vi "XY Graph Show-Hide Grid.vi"(8 "Error In":errorcluster, 9 "Hide (F) /Show (T)":bool, 11 "XYGraph Ref":T1) -> (0 "Error Out":errorcluster, 1 "Grid Shown?":bool, 3 "XYGraph Ref out":T1)   [LabVIEW 2021, in "XY Graph Add-Ons.lvlib"]
uses:
  XY Graph Add-Ons.lvlib
  XY Graph Refnum.ctl
  <vilib>/Utility/miscctls.llb/LVMajorAndMinorColorsTypeDef.ctl
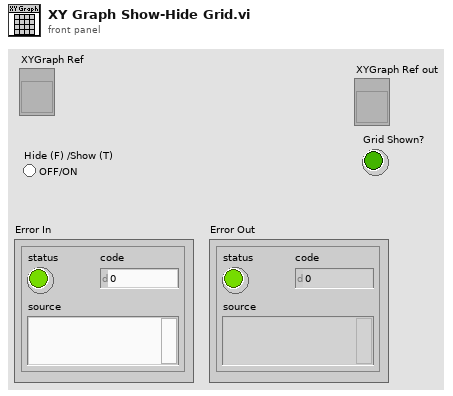
[diagram p1: front panel]
types:
  T1 = typedef "XY Graph Add-Ons.lvlib/XY Graph Refnum.ctl" = refnum<vi>
  T2 = typedef "LVMajorAndMinorColorsTypeDef.ctl" = cluster{"Major Color":u32, "Minor Color":u32}
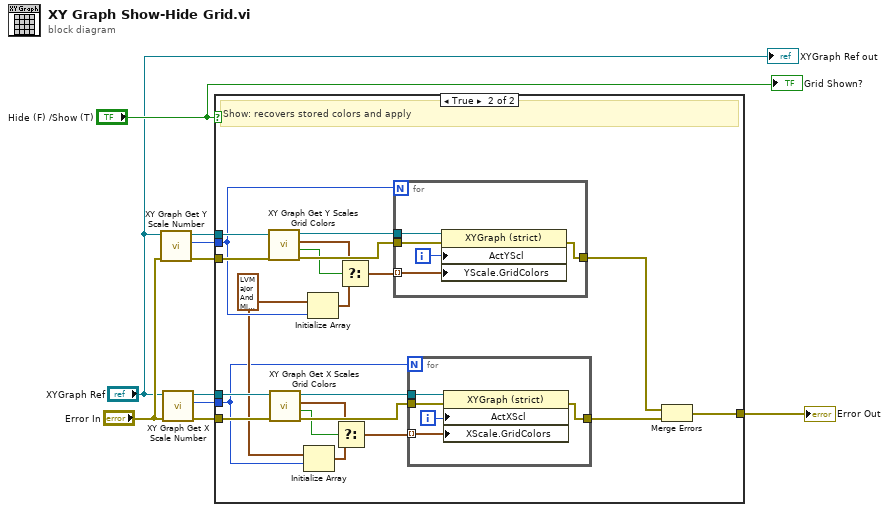
[diagram p0: block diagram]
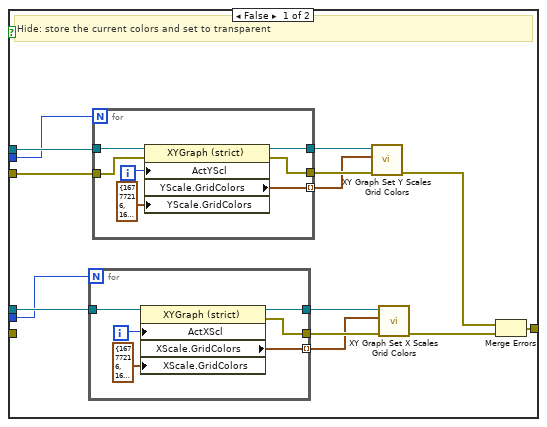
[diagram p2: hidden frame]
diagram:
  n1 = call "XY Graph Get Y Scale Number.vi"("Error In"="Error In", "XYGraph Ref"="XYGraph Ref") -> ("Error Out"=w3:errorcluster, "# Y Scales"=w2:i32, "XYGraph Ref out"=w4:T1)  [unwired: 7 in]
  n2 = call "XY Graph Get X Scale Number.vi"("Error In"="Error In", "XYGraph Ref"="XYGraph Ref") -> ("Error Out"=w7:errorcluster, "# X Scales"=w5:i32, "XYGraph Ref out"=w6:T1)  [unwired: 7 in]
  n3 = case shown="True" "Hide (F) /Show (T)" {
    tunnel: w6 -> [w24 w53]
    tunnel: [w16 w51] -> w10
    tunnel: w7 -> [_ w54]
    tunnel: w5 -> [w11 w39]
    tunnel: w4 -> [w14 w52]
    tunnel: w3 -> [w13 w49]
    tunnel: w2 -> [w12 w45]
    frame False {
      # "Hide: store the current colors and set to transparent"
      n4 = for {
        N: w11 -> [_]
        tunnel: [w34] -> w22 mode=indexing
        tunnel: [w36] -> w23
        tunnel: w24 -> [w37]
        tunnel: [w35] -> w21
        i -> [w32]
        n5 = property class="XYGraph (strict)"(reference=w37, "ActXScl"=w32, "XScale.GridColors"=cluster{"Major Color":u32, "Minor Color":u32} {"Major Color"=16777216, "Minor Color"=16777216} ("X Scale.Grid Colors")) -> (reference out=w35:T1, error out=w36:errorcluster, "XScale.GridColors"=w34:T2)  [unwired: 1 in]
      }
      n6 = for {
        N: w12 -> [_]
        tunnel: [w27] -> w18 mode=indexing
        tunnel: w13 -> [w30]
        tunnel: [w29] -> w19
        tunnel: w14 -> [w31]
        tunnel: [w28] -> w20
        i -> [w25]
        n7 = property class="XYGraph (strict)"(reference=w31, error in=w30, "ActYScl"=w25, "YScale.GridColors"=cluster{"Major Color":u32, "Minor Color":u32} {"Major Color"=16777216, "Minor Color"=16777216} ("X Scale.Grid Colors")) -> (reference out=w28:T1, error out=w29:errorcluster, "YScale.GridColors"=w27:T2)
      }
      n8 = call "XY Graph Set Y Scales Grid Colors.vi"("error in (no error)"=w19, "Array of Grid Colors"=w18, "XYGraph in"=w20) -> ("error out"=w17:errorcluster)  [unwired: 7 in, 1 out]
      n9 = call "XY Graph Set X Scales Grid Colors.vi"("error in (no error)"=w23, "Array of Grid Colors"=w22, "XYGraph in"=w21) -> ("error out"=w15:errorcluster)  [unwired: 7 in, 1 out]
      n10 = Merge Errors(w17, w15) -> (w16:errorcluster)
    }
    frame True {
      w40 = T2 {"Major Color"=13816530, "Minor Color"=13816530} ("Y Scale.Grid Colors")
      # "Show: recovers stored colors and apply"
      n11 = call "XY Graph Get Y Scales Grid Colors.vi"("error in (no error)"=w49, "XYGraph in"=w52) -> ("error out"=w56:errorcluster, "Was Tag Found?"=w48:bool, "Y Scale.Grid Colors"=w47:cluster{"Major Color":u32, "Minor Color":u32}[], "XYGraph out"=w55:T1)  [unwired: 6 in]
      n12 = call "XY Graph Get X Scales Grid Colors.vi"("error in (no error)"=w54, "XYGraph in"=w53) -> ("error out"=w59:errorcluster, "Was Tag Found?"=w43:bool, "X Scale.Grid Colors"=w42:cluster{"Major Color":u32, "Minor Color":u32}[], "XYGraph out"=w57:T1)  [unwired: 6 in]
      n13 = Initialize Array(w40, w39) -> (w38:T2[])
      n14 = Initialize Array(w40, w45) -> (w44:T2[])
      n15 = Select(t=w42, s=w43, f=w38) -> (s? t:f=w41:T2[])
      n16 = Select(t=w47, s=w48, f=w44) -> (s? t:f=w46:T2[])
      n17 = for {
        N: w45 -> [_]
        tunnel: [w68] -> w58
        tunnel: w56 -> [w67]
        tunnel: w46 -> [w66] mode=indexing
        tunnel: w55 -> [w69]
        i -> [w65]
        n18 = property class="XYGraph (strict)"(reference=w69, error in=w67, "ActYScl"=w65, "YScale.GridColors"=w66) -> (error out=w68:errorcluster)  [unwired: 1 out]
      }
      n19 = for {
        N: w39 -> [_]
        tunnel: [w63] -> w50
        tunnel: w59 -> [w62]
        tunnel: w41 -> [w61] mode=indexing
        tunnel: w57 -> [w64]
        i -> [w60]
        n20 = property class="XYGraph (strict)"(reference=w64, error in=w62, "ActXScl"=w60, "XScale.GridColors"=w61) -> (error out=w63:errorcluster)  [unwired: 1 out]
      }
      n21 = Merge Errors(w58, w50) -> (w51:errorcluster)
    }
  }
  "Error Out" <- w10
  "Grid Shown?" <- "Hide (F) /Show (T)"
  "XYGraph Ref out" <- "XYGraph Ref"
